vi "Return single characters from string.vi"(3 "Invert order?":bool, 4 "Input string":string, 5 "error in":errorcluster) -> (14 "Character array":string[](array[string]), 19 "error out":errorcluster)   [LabVIEW 2020]
doc: "Get single characters from input string."
panel:
  # "Get single characters from input string."
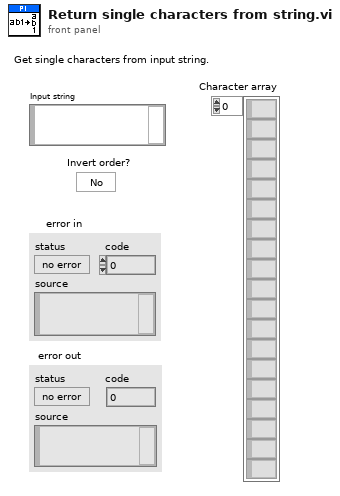
[diagram p1: front panel]
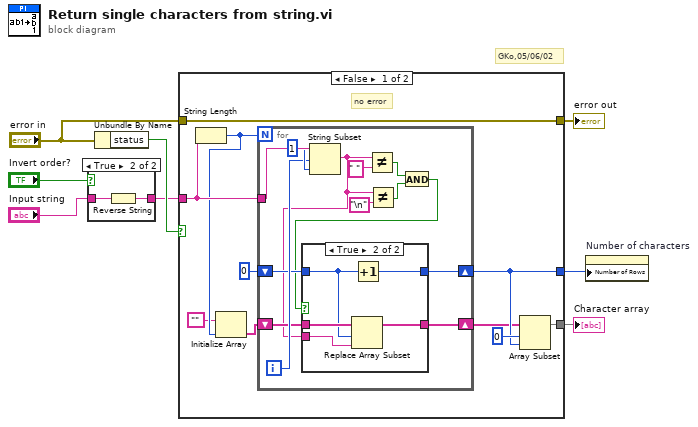
[diagram p0: block diagram]
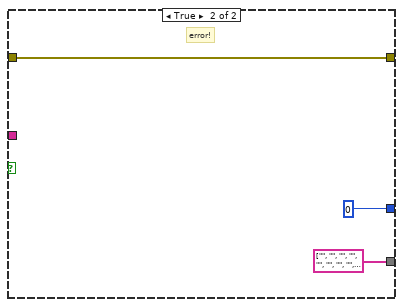
[diagram p4: hidden frame]
diagram:
  # "GKo,05/06/02"
  n1 = case shown="True" "Invert order?" {
    tunnel: "Input string" -> [w9 w11]
    tunnel: [w9 w10] -> w6
    frame False {
    }
    frame True {
      n2 = Reverse String(1:w11) -> (0:w10:string)
    }
  }
  n3 = Unbundle By Name("error in") -> ("status"=w8:bool)
  n4 = case shown="False" w8 {
    tunnel: w6 -> [w21 _]
    tunnel: [w15 0] -> w5
    tunnel: [w13 string[] ["", "", "", "", "", "", "", "", "", "", "", "", "", "", "", "", "", "", "", "", "", "", "", "", "", "", ""] ("Conn. Axes 2")] -> w4
    tunnel: [w12 w42] -> w2
    tunnel: "error in" -> [w12 w42]
    frame False {
      # "no error"
      n5 = String Length(string=w21) -> (length=w19:i32)
      n6 = Initialize Array("" ("Element Data"), w19) -> (w17:string[])
      n7 = for {
        N: w19 -> [_]
        tunnel: w21 -> [w34]
        shift-right: [w27] -> w14
        shift-left: w17 -> [w28]
        shift-right: [w30] -> w15
        shift-left: 0 -> [w29]
        i -> [w32]
        n8 = String Subset(string=w34, offset (0)=w32, length (rest)=1 ("length")) -> (substring=w26:string)
        n9 = Not Equal?(x=w26, y=" ") -> (x != y?=w24:bool)
        n10 = Not Equal?(x=w26, y="\n") -> (x != y?=w23:bool)
        n11 = And(x=w24, y=w23) -> (x .and. y?=w22:bool)
        n12 = case shown="True" w22 {
          tunnel: [w36 w41] -> w30
          tunnel: w29 -> [w36 w39]
          tunnel: w28 -> [w35 w40]
          tunnel: w26 -> [_ w38]
          tunnel: [w35 w37] -> w27
          frame False {
          }
          frame True {
            n13 = Replace Array Subset(array=w40, new element=w38, index=w39) -> (w37:string[])
            n14 = Increment(x=w39) -> (x+1=w41:i32)
          }
        }
      }
      n15 = Array Subset(array=w14, index=0 ("Array Index"), length=w15) -> (w13:string[])
    }
    frame True {
      # "error!"
    }
  }
  "error out" <- w2
  "Character array" <- w4
  n16 = property on="Number of characters" class="Arr (strict)"("Number of Rows"=w5) -> ()  [unwired: 2 in, 2 out]
